vi "PulseTrain-Init (Continuous).vi"(0 "Pulse Train Params":T2, 5 "Start Pulse Rate (Hz)":dbl, 7 "Start Phase (cycles)":dbl, 9 "Fs (Hz)":dbl, 11 "error in (no error)":errorcluster) -> (4 "Initial State":T1, 15 "error out":errorcluster)   [LabVIEW 2020]
uses:
  Pulse Train Params.ctl
  Pulse Polarity.ctl
  PT-Continuous State.ctl
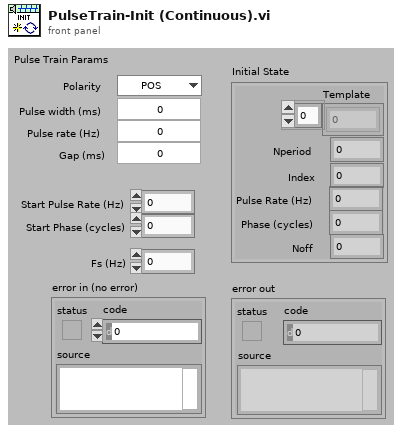
[diagram p1: front panel]
types:
  T1 = typedef "PT-Continuous State.ctl" = cluster{"Template":dbl[], "Nperiod":i32, "Index":i32, "Pulse Rate (Hz)":dbl, "Phase (cycles)":dbl, "Noff":i32}
  T2 = typedef "Pulse Train Params.ctl" = cluster{"Pulse width (us)":dbl, "Pulse rate (Hz)":dbl, "Gap (ms)":dbl, "Polarity":T3, "PT State":T1, "Asynch":bool}
  T3 = typedef "Pulse Polarity.ctl" = enum16{"POS", "NEG", "POS-NEG", "NEG-POS"}
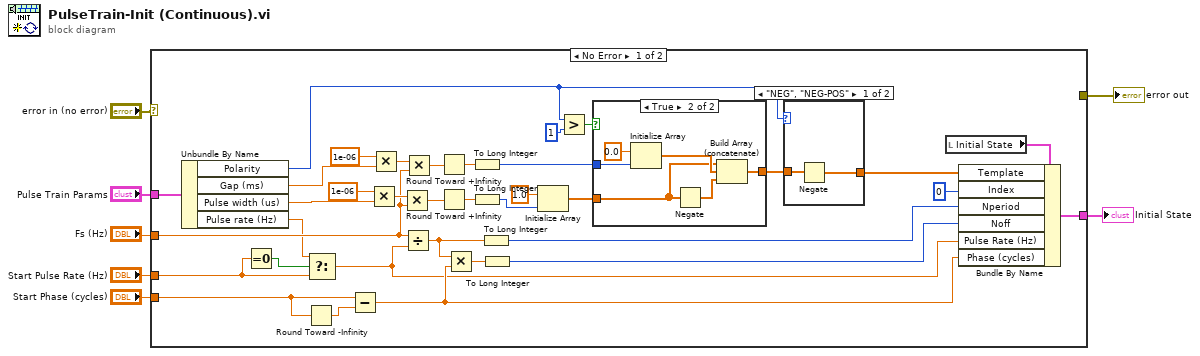
[diagram p0: block diagram]
diagram:
  n1 = case shown="No Error" "error in (no error)" {
    selector: "error in (no error)" -> [_ w53]
    tunnel: [_ w53] -> w6
    tunnel: "Pulse Train Params" -> [w24 _]
    tunnel: "Fs (Hz)" -> [w20 _]
    tunnel: [w21 _] -> w3
    tunnel: "Start Pulse Rate (Hz)" -> [w10 _]
    tunnel: "Start Phase (cycles)" -> [w12 _]
    frame No Error {
      n2 = Unbundle By Name(w24) -> ("Polarity"=w26:T3, "Gap (ms)"=w33:dbl, "Pulse width (us)"=w42:dbl, "Pulse rate (Hz)"=w8:dbl)
      n3 = Equal To 0?(x=w10) -> (x = 0?=w11:bool)
      n4 = Round Toward -Infinity(1:w12) -> (0:w13:dbl)
      n5 = Select(t=w8, s=w11, f=w10) -> (s? t:f=w9:dbl)
      n6 = Subtract(x=w12, y=w13) -> (x-y=w14:dbl)
      n7 = Multiply(x=1e-06, y=w42) -> (x*y=w40:dbl)
      n8 = Multiply(x=1e-06, y=w33) -> (x*y=w34:dbl)
      n9 = Multiply(x=w40, y=w20) -> (x*y=w39:dbl)
      n10 = Divide(x=w20, y=w9) -> (x/y=w16:dbl)
      n11 = Multiply(x=w34, y=w20) -> (x*y=w31:dbl)
      n12 = Round Toward +Infinity(x=w31) -> (ceil(x): smallest int >= x=w32:dbl)
      n13 = Round Toward +Infinity(x=w39) -> (ceil(x): smallest int >= x=w38:dbl)
      n14 = Multiply(x=w16, y=w14) -> (x*y=w19:dbl)
      n15 = To Long Integer(number=w32) -> (32bit integer=w27:i32)
      n16 = To Long Integer(number=w38) -> (32bit integer=w37:i32)
      n17 = To Long Integer(number=w16) -> (32bit integer=w15:i32)
      n18 = To Long Integer(number=w19) -> (32bit integer=w17:i32)
      n19 = Initialize Array(1.0 ("element"), w37) -> (w28:dbl[])
      n20 = Greater?(x=w26, y=u16 1) -> (0:w30:bool)
      n21 = case shown="True" w30 {
        tunnel: w28 -> [w46 w49]
        tunnel: w27 -> [_ w52]
        tunnel: [w46 w47] -> w25
        frame False {
        }
        frame True {
          n22 = Initialize Array(0.0 ("element"), w52) -> (w50:dbl[])
          n23 = Negate(x=w49) -> (-x=w48:dbl[])
          n24 = Build Array (concatenate)(w49, w50, w48) -> (w47:dbl[])
        }
      }
      n25 = case shown="\"NEG\", \"NEG-POS\"" w26 {
        tunnel: w25 -> [w44 w45]
        tunnel: [w43 w45] -> w22
        frame "NEG", "NEG-POS" {
          n26 = Negate(x=w44) -> (-x=w43:dbl[])
        }
        frame "POS", "POS-NEG", Default {
        }
      }
      n27 = local read "Initial State"() -> (w23:T1)
      n28 = Bundle By Name(cluster=w23, "Template"=w22, "Index"=0, "Nperiod"=w15, "Noff"=w17, "Pulse Rate (Hz)"=w9, "Phase (cycles)"=w14) -> (w21:T1)
    }
    frame Error {
    }
  }
  "error out" <- w6
  "Initial State" <- w3
